vi "read default menu name.vi"(8 "error in":errorcluster, 11 "EthernetIP editor node in":refnum<class "EIP Tags editor node.lvclass">) -> (0 "error out":errorcluster, 2 "default menu name":string, 3 "EthernetIP editor node out":refnum<class "EIP Tags editor node.lvclass">)   [LabVIEW 2013, in "EIP Tags editor node.lvclass"]
uses:
  EIP Tags editor node.lvclass
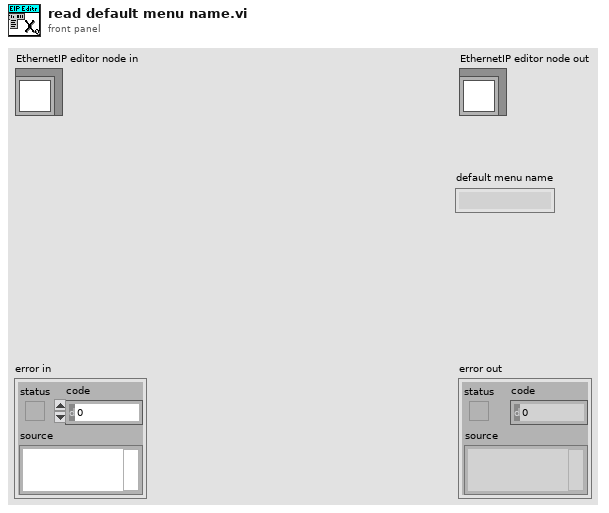
[diagram p1: front panel]
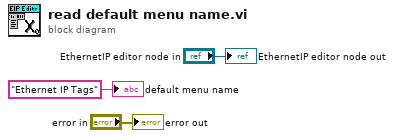
[diagram p0: block diagram]
diagram:
  "error out" <- "error in"
  "EthernetIP editor node out" <- "EthernetIP editor node in"
  "default menu name" <- "Ethernet IP Tags" ("default menu name")
